vi "TLC Main.vi"(8 "error in (no error)":errorcluster) -> (0 "error out":errorcluster)   [LabVIEW 2009]
doc: "[Covers: REQ_UserInterface]\nThis is the main user interface for the Theatre Light Control Software.\n\n[Covers: REQ_UserInterfaceMenu]\nSystem uses tlc_Menu.mnu to implement the menu. Verify with Edit»Run-Time Menu.\n\n[Covers: REQ_SoftwareResponseRequirement]\nThe application uses the Producer/Consumer with Events Design pattern to guarantee that the execution occurs within 100ms.\n\n[Covers: REQ_SystemResponseRequirement]\nThe system loops are dependent on an event being generated, which maintains the CPU usage requirement.\n\n[Covers: REQ_Stop]\nFlushes the queue and stops execution of the cue list if the user clicks on the Stop button."
uses:
  Controls/tlc_Cue_Information.ctl
  Controls/channel.ctl
  Controls/tlc_Consumer Control.ctl
  Controls/tlc_Functions.ctl
  Controls/tlc_User Interface Command.ctl
  Controls/tlc_User Interface Data Type.ctl
  Modules/Error/tlc_Error Module Command Control.ctl
  Instance          14 16Saved   TLC Main .vi
  Instance          15 16Saved   TLC Main .vi
  Modules/File/tlc_File_Command Control.ctl
  Modules/Cue/tlc_Cue_Information Command.ctl
panel:
  out "Cue Information":T1 {"Channels"."Intensity" min=0.0 max=100.0 step=1.0 format="%#.0f"}
  in  "Stop":bool
  in  "Record":bool
  in  "Play":bool
  out "Cue List":i32(listbox)
  # "Cue Control"
  # "Cue Information"
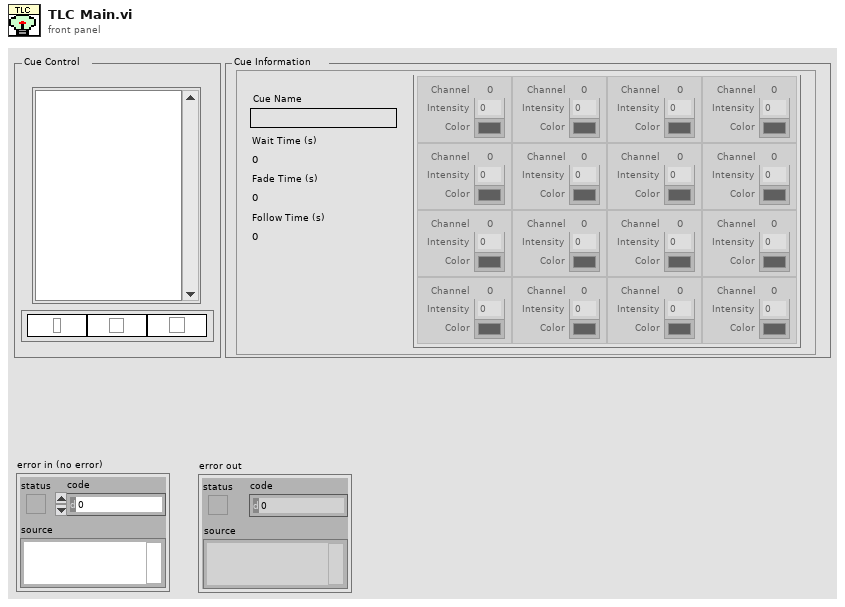
[diagram p1: front panel]
types:
  T1 = typedef "tlc_Cue_Information.ctl" = cluster{"Cue Name":string, "Wait Time (s)":u32, "Fade Time (s)":u32, "Follow Time (s)":u32, "Channels":T2[][]}
  T2 = typedef "channel.ctl" = cluster{"Intensity":dbl, " Color":u32, "Channel":i32}
  T3 = typedef "tlc_Error Module Command Control.ctl" = enum16{"Initialize", "Handle Errors", "Report Errors"}
  T4 = typedef "tlc_User Interface Command.ctl" = cluster{"Data Type":T5, "Data":variant}
  T5 = typedef "tlc_User Interface Data Type.ctl" = enum16{"Initialize", "Initialize Front Panel", "Update Front Panel Channels", "Select Cue in Cue List", "Enable/Disable Front Panel Controls", "Update Cue List", "Stop"}
  T6 = typedef "tlc_Consumer Control.ctl" = cluster{"Command":T7, "Data":variant}
  T7 = typedef "tlc_Functions.ctl" = enum16{"Initialize", "Record", "Load", "Save", "Play", "Stop", "Exit"}
  T8 = typedef "tlc_Cue_Information Command.ctl" = enum16{"Add Cue", "Get Cue Values", "Set Cue Values", "Get Number of Cues", "Initialize", "Get Empty Cue"}
  T9 = typedef "tlc_File_Command Control.ctl" = enum16{"Initialize", "Save Cues", "Load Cues", "Shutdown"}
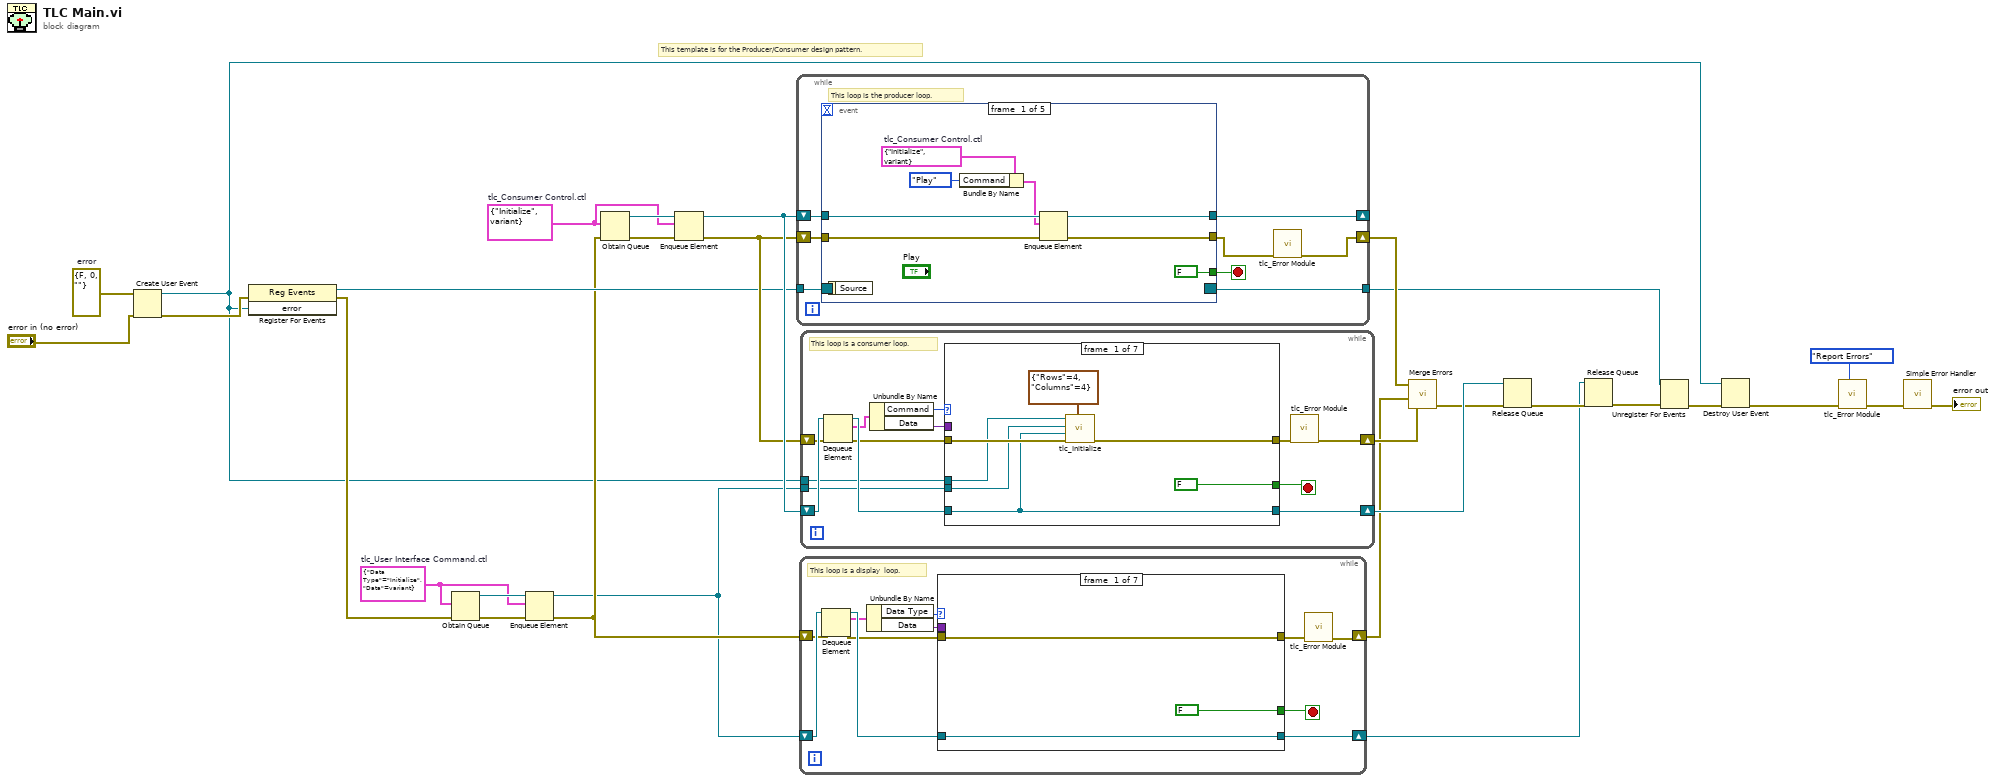
[diagram p0: block diagram]
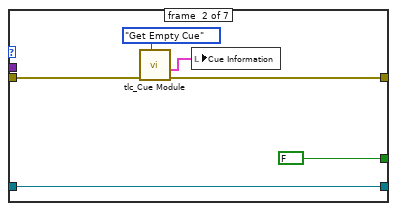
[diagram p2: hidden frame]
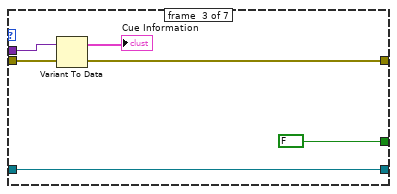
[diagram p3: hidden frame]
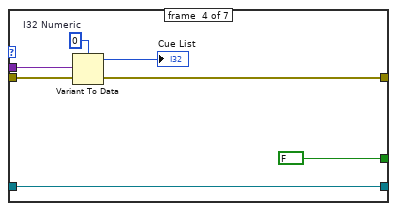
[diagram p4: hidden frame]
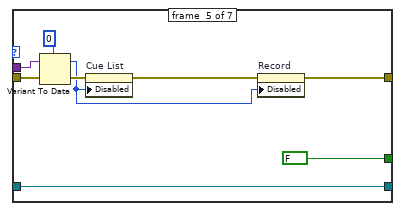
[diagram p5: hidden frame]
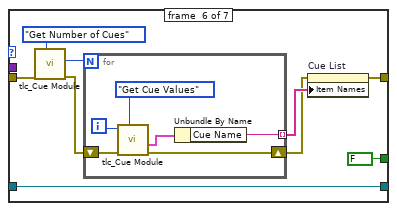
[diagram p6: hidden frame]
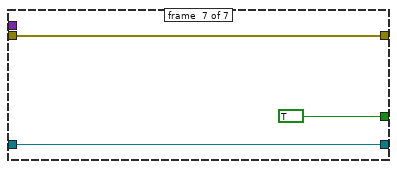
[diagram p7: hidden frame]
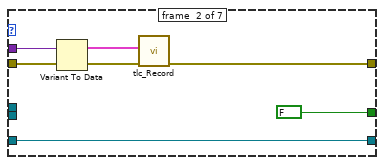
[diagram p8: hidden frame]
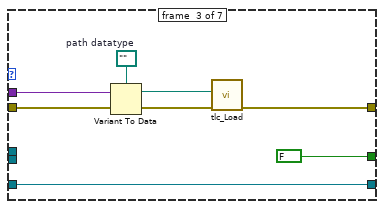
[diagram p9: hidden frame]
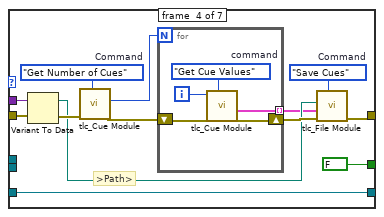
[diagram p10: hidden frame]
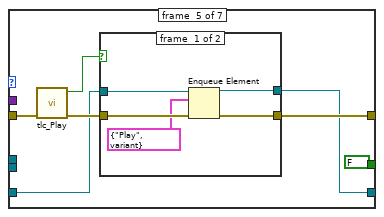
[diagram p11: hidden frame]
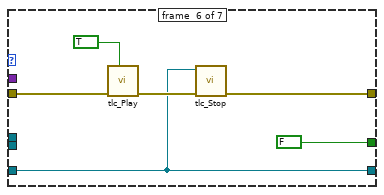
[diagram p13: hidden frame]
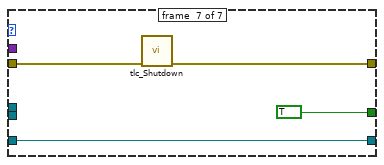
[diagram p14: hidden frame]
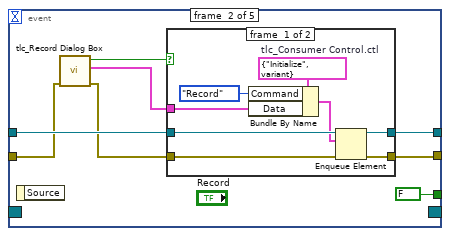
[diagram p15: hidden frame]
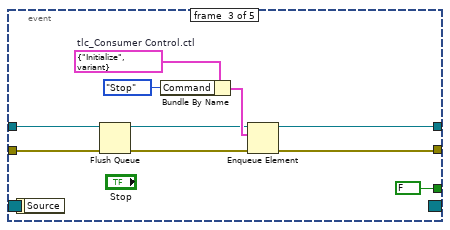
[diagram p17: hidden frame]
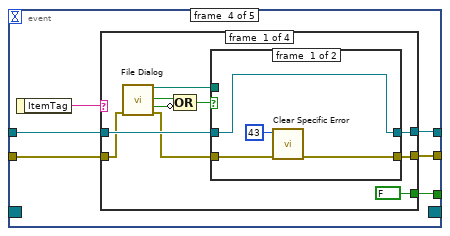
[diagram p18: hidden frame]
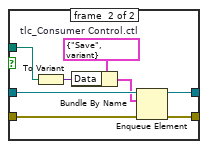
[diagram p19: hidden frame]
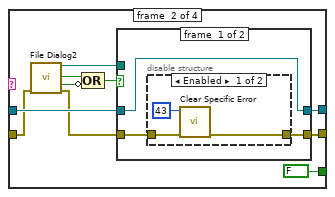
[diagram p20: hidden frame]
diagram:
  w13 = T4 {"Data Type"=enum."Initialize", "Data"=variant}  # tlc_User Interface Command.ctl
  w25 = errorcluster {"status"=FALSE, "code"=0, "source"=""}  # error
  w27 = T6 {"Command"=enum."Initialize", "Data"=variant}  # tlc_Consumer Control.ctl
  # "This template is for the Producer/Consumer design pattern."
  n1 = Create User Event(user event datatype=w25, error in="error in (no error)") -> (user event=w7:refnum<user-event>, error out=w24:errorcluster)
  n2 = register-events(error in=w24, w7) -> (reference out=w23:refnum<event-registration>, error out=w12:errorcluster)  [unwired: 1 in]
  n3 = Obtain Queue(element data type=w13, error in (no error)=w12) -> (queue out=w15:refnum<queue>, error out=w14:errorcluster)  [unwired: 2 in, 2 out]
  n4 = Enqueue Element(queue=w15, element=w13, error in (no error)=w14) -> (queue out=w6:refnum<queue>, error out=w11:errorcluster)  [unwired: 2 out]
  n5 = Obtain Queue(element data type=w27, error in (no error)=w11) -> (queue out=w30:refnum<queue>, error out=w29:errorcluster)  [unwired: 2 in, 2 out]
  n6 = Enqueue Element(queue=w30, element=w27, error in (no error)=w29) -> (queue out=w28:refnum<queue>, error out=w26:errorcluster)  [unwired: 2 out]
  n7 = while {
    shift-right: [w31] -> w20
    shift-left: w26 -> [w37]
    shift-right: [w35] -> _
    shift-left: w28 -> [w38]
    tunnel: w23 -> [w34]
    tunnel: [w33] -> w17
    stop <- w36 stop-if-true
    # "This loop is the producer loop."
    n8 = event shown="[2] \"Stop\": Value Change" {
      selector: w34 -> [_ _ _ _ _]
      dyn-events: [_ _ _ _ _] -> w33
      timeout: _ -> [_ _ _ _ _]
      tunnel: w38 -> [w45 w53 w73 w79 w139]
      tunnel: w37 -> [w44 w48 w69 w78 w138]
      tunnel: [w43 w52 w65 w76 w138] -> w32
      tunnel: [FALSE FALSE FALSE w75 w140] -> w36
      tunnel: [w39 w51 w66 w77 w139] -> w35
      event #0 {
        w42 = T6 {"Command"=enum."Initialize", "Data"=variant}  # tlc_Consumer Control.ctl
        n9 = event-data() -> ()  [unwired: 2 out]
        n10 = Bundle By Name(cluster=w42, "Command"=tlc_Functions."Play") -> (w41:T6)
        n11 = Enqueue Element(queue=w45, element=w41, error in (no error)=w44) -> (queue out=w39:refnum<queue>, error out=w43:errorcluster)  [unwired: 2 out]
      }
      event #1 {
        n12 = event-data() -> ()  [unwired: 2 out]
        n13 = call "tlc_Record Dialog Box.vi"("error in (no error)"=w48) -> ("error out"=w47:errorcluster, "Output Cue"=w49:T1, "Cancelled?"=w50:bool)  [unwired: 8 out]
        n14 = case shown="False" w50 {
          tunnel: w53 -> [w62 w64]
          tunnel: w47 -> [w61 w63]
          tunnel: [w60 w63] -> w52
          tunnel: [w56 w64] -> w51
          tunnel: w49 -> [w55 _]
          frame #0 {
            w59 = T6 {"Command"=enum."Initialize", "Data"=variant}  # tlc_Consumer Control.ctl
            n15 = Bundle By Name(cluster=w59, "Command"=tlc_Functions."Record", "Data"=w55) -> (w58:T6)
            n16 = Enqueue Element(queue=w62, element=w58, error in (no error)=w61) -> (queue out=w56:refnum<queue>, error out=w60:errorcluster)  [unwired: 2 out]
          }
          frame #1 {
          }
        }
      }
      event #2 {
        w72 = T6 {"Command"=enum."Initialize", "Data"=variant}  # tlc_Consumer Control.ctl
        n17 = event-data() -> ()  [unwired: 2 out]
        n18 = Flush Queue(queue=w73, error in (no error)=w69) -> (queue out=w67:refnum<queue>, error out=w68:errorcluster)  [unwired: 1 out]
        n19 = Bundle By Name(cluster=w72, "Command"=tlc_Functions."Stop") -> (w71:T6)
        n20 = Enqueue Element(queue=w67, element=w71, error in (no error)=w68) -> (queue out=w66:refnum<queue>, error out=w65:errorcluster)  [unwired: 2 out]
      }
      event #3 {
        n21 = event-data() -> ("ItemTag"=w80:string)  [unwired: 1 out]
        n22 = case shown="Default" w80 {
          tunnel: w79 -> [w85 w107 w134 w137]
          tunnel: w78 -> [w82 w104 w132 w136]
          tunnel: [w84 w106 w133 w137] -> w77
          tunnel: [w83 w105 w131 w136] -> w76
          tunnel: [FALSE FALSE TRUE FALSE] -> w75
          frame #0 {
            n23 = call "File Dialog"("error in"=w82) -> ("selected path"=w86:path, "exists"=w88:bool, "cancelled"=w89:bool, "error out"=w81:errorcluster)  [unwired: 6 in, 5 out]
            n24 = Compound Arithmetic op=OR(w88, invert w89) -> (w87:bool)
            n25 = case shown="False" w87 {
              tunnel: w86 -> [_ w95]
              tunnel: w85 -> [w94 w102]
              tunnel: w81 -> [w93 w101]
              tunnel: [w94 w100] -> w84
              tunnel: [w92 w99] -> w83
              frame #0 {
                n26 = call "Clear Specific Error.vi"("error in (no error)"=w93, "Code"=43) -> ("error out"=w92:errorcluster)  [unwired: 5 out]
              }
              frame #1 {
                w98 = T6 {"Command"=enum."Save", "Data"=variant}  # tlc_Consumer Control.ctl
                n27 = To Variant(anything=w95) -> (Variant=w96:variant)
                n28 = Bundle By Name(cluster=w98, "Data"=w96) -> (w97:T6)
                n29 = Enqueue Element(queue=w102, element=w97, error in (no error)=w101) -> (queue out=w100:refnum<queue>, error out=w99:errorcluster)  [unwired: 2 out]
              }
            }
          }
          frame #1 {
            n30 = call "File Dialog2"("error in"=w104) -> ("selected path"=w108:path, "exists"=w110:bool, "cancelled"=w111:bool, "error out"=w103:errorcluster)  [unwired: 6 in, 5 out]
            n31 = Compound Arithmetic op=OR(w110, invert w111) -> (w109:bool)
            n32 = case shown="True" w109 {
              tunnel: w108 -> [_ w119]
              tunnel: w107 -> [w115 w126]
              tunnel: w103 -> [w114 w125]
              tunnel: [w115 w124] -> w106
              tunnel: [w113 w123] -> w105
              frame #0 {
                n33 = disable-structure shown="Enabled" {
                  disable-tunnel: w114 -> [w117 _]
                  disable-tunnel: [w116 _] -> w113
                  frame #0 {
                    n34 = call "Clear Specific Error.vi"("error in (no error)"=w117, "Code"=43) -> ("error out"=w116:errorcluster)  [unwired: 5 out]
                  }
                  frame #1 {
                  }
                }
              }
              frame #1 {
                w122 = T6 {"Command"=enum."Load", "Data"=variant}  # tlc_Consumer Control.ctl
                n35 = To Variant(anything=w119) -> (Variant=w120:variant)
                n36 = Bundle By Name(cluster=w122, "Data"=w120) -> (w121:T6)
                n37 = Enqueue Element(queue=w126, element=w121, error in (no error)=w125) -> (queue out=w124:refnum<queue>, error out=w123:errorcluster)  [unwired: 2 out]
              }
            }
          }
          frame #2 {
            w130 = T6 {"Command"=enum."Initialize", "Data"=variant}  # tlc_Consumer Control.ctl
            n38 = Bundle By Name(cluster=w130, "Command"=tlc_Functions."Exit") -> (w127:T6)
            n39 = Enqueue Element(queue=w134, element=w127, error in (no error)=w132) -> (queue out=w133:refnum<queue>, error out=w131:errorcluster)  [unwired: 2 out]
          }
          frame #3 {
          }
        }
      }
      event #4 {
        n40 = event-data() -> ("status"=w140:bool)  [unwired: 1 out]
      }
    }
    n41 = call "tlc_Error Module.vi"("error in (no error)"=w32) -> ("error out"=w31:errorcluster)  [unwired: 4 in, 6 out]
  }
  n42 = while {
    shift-right: [w149] -> w9
    shift-left: w6 -> [w151]
    shift-right: [w141] -> w5
    shift-left: w11 -> [w148]
    stop <- w144 stop-if-true
    # "This loop is a display  loop."
    n43 = Dequeue Element(queue=w151, error in (no error)=w148) -> (queue out=w150:refnum<queue>, element=w147:T4, error out=w145:errorcluster)  [unwired: 2 out]
    n44 = Unbundle By Name(w147) -> ("Data Type"=w146:T5, "Data"=w143:variant)
    n45 = case shown="\"Initialize\", Default" w146 {
      tunnel: w150 -> [w154 w160 w166 w173 w182 w191 w199]
      tunnel: [w154 w160 w166 w173 w182 w191 w199] -> w149
      tunnel: w145 -> [w153 w158 w163 w170 w179 w189 w200]
      tunnel: [w153 w157 w161 w169 w174 w185 w200] -> w142
      tunnel: [FALSE FALSE FALSE FALSE FALSE FALSE TRUE] -> w144
      tunnel: w143 -> [_ _ w164 w171 w180 _ _]
      frame #0 {
      }
      frame #1 {
        n46 = call "tlc_Cue Module.vi"("Command"=tlc_Cue_Information_Command."Get Empty Cue", "error in (no error)"=w158) -> ("error out"=w157:errorcluster, "Cue Output"=w155:T1)  [unwired: 3 in, 4 out]
        n47 = local write "Cue Information"(w155) -> ()
      }
      frame #2 {
        n48 = Variant To Data(error in=w163, Variant=w164) -> (error out=w161:errorcluster, data=→"Cue Information":T1)  [unwired: 1 out]
      }
      frame #3 {
        w167 = 0  # I32 Numeric
        n49 = Variant To Data(error in=w170, Variant=w171, type=w167) -> (error out=w169:errorcluster, data=→"Cue List":i32)
      }
      frame #4 {
        n50 = Variant To Data(error in=w179, Variant=w180, type=u8 0) -> (error out=w177:errorcluster, data=w176:u8)
        n51 = property on="Cue List" class="LstBox (strict)"(error in=w177, "Disabled"=w176) -> (error out=w175:errorcluster)  [unwired: 1 in, 1 out]
        n52 = property on="Record" class="Bool"(error in=w175, "Disabled"=w176) -> (error out=w174:errorcluster)  [unwired: 1 in, 1 out]
      }
      frame #5 {
        n53 = call "tlc_Cue Module.vi"("Command"=tlc_Cue_Information_Command."Get Number of Cues", "error in (no error)"=w189) -> ("error out"=w186:errorcluster, "Number of Cues"=w187:i32)  [unwired: 3 in, 4 out]
        n54 = for {
          N: w187 -> [_]
          shift-right: [w196] -> w183
          shift-left: w186 -> [w197]
          tunnel: [w192] -> w184 mode=indexing
          i -> [w194]
          n55 = call "tlc_Cue Module.vi"("Command"=tlc_Cue_Information_Command."Get Cue Values", "error in (no error)"=w197, "Cue Index"=w194) -> ("error out"=w196:errorcluster, "Cue Output"=w193:T1)  [unwired: 2 in, 4 out]
          n56 = Unbundle By Name(w193) -> ("Cue Name"=w192:string)
        }
        n57 = property on="Cue List" class="LstBox (strict)"(error in=w183, "Item Names"=w184) -> (error out=w185:errorcluster)  [unwired: 1 in, 1 out]
      }
      frame #6 {
      }
    }
    n58 = call "tlc_Error Module.vi"("error in (no error)"=w142) -> ("error out"=w141:errorcluster)  [unwired: 4 in, 6 out]
  }
  n59 = while {
    shift-right: [w211] -> w19
    shift-left: w28 -> [w213]
    shift-right: [w201] -> w21
    shift-left: w26 -> [w210]
    tunnel: w7 -> [w204]
    tunnel: w6 -> [w203]
    stop <- w206 stop-if-true
    # "This loop is a consumer loop."
    n60 = Dequeue Element(queue=w213, error in (no error)=w210) -> (queue out=w212:refnum<queue>, element=w209:T6, error out=w207:errorcluster)  [unwired: 2 out]
    n61 = Unbundle By Name(w209) -> ("Command"=w208:T7, "Data"=w205:variant)
    n62 = case shown="\"Stop\"" w208 {
      tunnel: w212 -> [w214 w227 w235 w248 w256 w268 w277]
      tunnel: [w214 w227 w235 w248 w254 w268 w277] -> w211
      tunnel: w207 -> [w219 w224 w232 w245 w259 w270 w275]
      tunnel: [w218 w221 w229 w239 w255 w272 w274] -> w202
      tunnel: [FALSE FALSE FALSE FALSE FALSE FALSE TRUE] -> w206
      tunnel: w205 -> [_ w225 w233 w246 _ _ _]
      tunnel: w204 -> [w216 _ _ _ _ _ _]
      tunnel: w203 -> [w215 _ _ _ _ _ _]
      frame #0 {
        n63 = call "tlc_Initialize.vi"("Number of Channels"=cluster{"Rows":i32, "Columns":i32} {"Rows"=4, "Columns"=4}, "error in (no error)"=w219, "tlc_Consumer Queue Reference.ctl"=w214, "tlc_Display Queue Reference.ctl"=w215, "tlc_User Event Reference.ctl"=w216) -> ("error out"=w218:errorcluster)  [unwired: 1 in, 5 out]
      }
      frame #1 {
        n64 = Variant To Data(error in=w224, Variant=w225) -> (error out=w223:errorcluster, data=w222:T1)  [unwired: 1 out]
        n65 = call "tlc_Record.vi"("error in (no error)"=w223, "Cue"=w222) -> ("error out"=w221:errorcluster)  [unwired: 9 out]
      }
      frame #2 {
        w228 = path ""  # path datatype
        n66 = Variant To Data(error in=w232, Variant=w233, type=w228) -> (error out=w231:errorcluster, data=w230:path)
        n67 = call "tlc_Load.vi"("error in (no error)"=w231, "Path"=w230) -> ("error out"=w229:errorcluster)  [unwired: 9 out]
      }
      frame #3 {
        w236 = tlc_File_Command_Control."Save Cues"  # Command
        w243 = tlc_Cue_Information_Command."Get Number of Cues"  # Command
        # ">Path>"
        n68 = Variant To Data(error in=w245, Variant=w246) -> (error out=w244:errorcluster, data=w238:path)  [unwired: 1 out]
        n69 = call "tlc_Cue Module.vi"("Command"=w243, "error in (no error)"=w244) -> ("error out"=w241:errorcluster, "Number of Cues"=w242:i32)  [unwired: 3 in, 4 out]
        n70 = for {
          N: w242 -> [_]
          tunnel: [w250] -> w237 mode=indexing
          shift-right: [w249] -> w240
          shift-left: w241 -> [w253]
          i -> [w251]
          w252 = tlc_Cue_Information_Command."Get Cue Values"  # command
          n71 = call "tlc_Cue Module.vi"("Command"=w252, "error in (no error)"=w253, "Cue Index"=w251) -> ("error out"=w249:errorcluster, "Cue Output"=w250:T1)  [unwired: 2 in, 4 out]
        }
        n72 = call "tlc_File Module.vi"("Command"=w236, "error in (no error)"=w240, "Cue Array Input"=w237, "Path"=w238) -> ("error out"=w239:errorcluster)  [unwired: 7 out]
      }
      frame #4 {
        n73 = call "tlc_Play.vi"("error in (no error)"=w259) -> ("error out"=w257:errorcluster, "Stop?"=w258:bool)  [unwired: 1 in, 8 out]
        n74 = case shown="False" w258 {
          tunnel: w257 -> [w264 w266]
          tunnel: w256 -> [w265 w267]
          tunnel: [w263 w266] -> w255
          tunnel: [w262 w267] -> w254
          frame #0 {
            n75 = Enqueue Element(queue=w265, element=T6 {"Command"=enum."Play", "Data"=variant}, error in (no error)=w264) -> (queue out=w262:refnum<queue>, error out=w263:errorcluster)  [unwired: 2 out]
          }
          frame #1 {
          }
        }
      }
      frame #5 {
        n76 = call "tlc_Play.vi"("Reset"=TRUE, "error in (no error)"=w270) -> ("error out"=w271:errorcluster)  [unwired: 9 out]
        n77 = call "tlc_Stop.vi"("error in"=w271, "tlc_Consumer Queue Reference.ctl"=w268) -> ("error out"=w272:errorcluster)  [unwired: 9 out]
      }
      frame #6 {
        n78 = call "tlc_Shutdown.vi"("error in (no error)"=w275) -> ("error out"=w274:errorcluster)  [unwired: 10 out]
      }
    }
    n79 = call "tlc_Error Module.vi"("error in (no error)"=w202) -> ("error out"=w201:errorcluster)  [unwired: 4 in, 6 out]
  }
  n80 = call <vilib>:"Merge Errors.vi"("error in 3 (no error)"=w5, "error in 2 (no error)"=w21, "error in 1 (no error)"=w20) -> ("error out"=w18:errorcluster)  [unwired: 1 in, 3 out]
  n81 = Release Queue(queue=w19, error in (no error)=w18) -> (error out=w10:errorcluster)  [unwired: 3 out]
  n82 = Release Queue(queue=w9, error in (no error)=w10) -> (error out=w8:errorcluster)  [unwired: 3 out]
  n83 = Unregister For Events(event registration refnum=w17, error in=w8) -> (error out=w16:errorcluster)
  n84 = Destroy User Event(user event=w7, error in=w16) -> (error out=w4:errorcluster)
  n85 = call "tlc_Error Module.vi"("Command (Handle Errors"=tlc_Error_Module_Command_Control."Report Errors", "error in (no error)"=w4) -> ("error out"=w3:errorcluster)  [unwired: 3 in, 6 out]
  n86 = call <vilib>:"Simple Error Handler.vi"("error in (no error)"=w3) -> ("error out"=→"error out":errorcluster)  [unwired: 1 in, 7 out]
